vi "B.vi"(10 "Array":string[](array[string]), 11 "String":string) -> (3 "B":string)   [LabVIEW 2017]
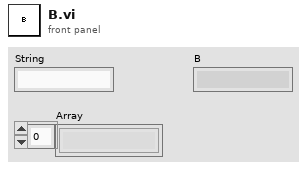
[diagram p1: front panel]
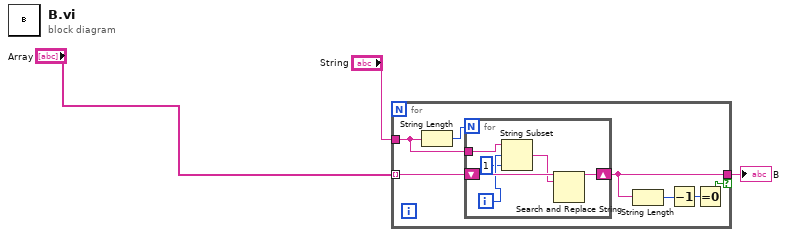
[diagram p0: block diagram]
diagram:
  n1 = for {
    tunnel: "Array" -> [w9] mode=indexing
    tunnel: "String" -> [w8]
    tunnel: [w6] -> w3 if=w4
    n2 = String Length(string=w8) -> (length=w10:i32)
    n3 = for {
      N: w10 -> [_]
      tunnel: w8 -> [w15]
      shift-right: [w11] -> w6
      shift-left: w9 -> [w16]
      i -> [w14]
      n4 = String Subset(string=w15, offset (0)=w14, length (rest)=1 ("length (rest)")) -> (substring=w12:string)
      n5 = Search and Replace String(input string=w16, search string=w12) -> (result string=w11:string)  [unwired: 6 in, 3 out]
    }
    n6 = String Length(string=w6) -> (length=w7:i32)
    n7 = Decrement(x=w7) -> (x-1=w5:i32)
    n8 = Equal To 0?(x=w5) -> (x = 0?=w4:bool)
  }
  "B" <- w3
